vi "S3859061_Task4.vi"() -> ()   [LabVIEW 2020]
panel:
  out "String":string
  in  "Enum 2":enum16{"Pizza", "Fries", "Noodle"}(ring)
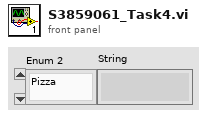
[diagram p1: front panel]
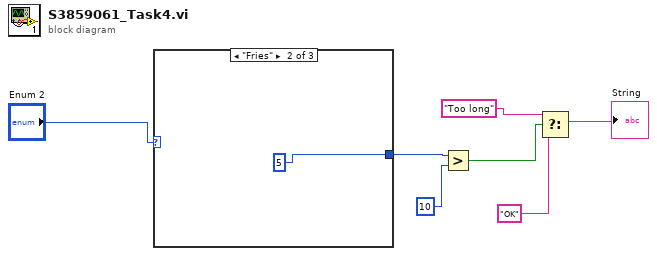
[diagram p0: block diagram]
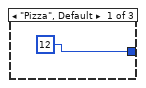
[diagram p2: hidden frame]
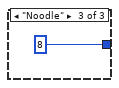
[diagram p3: hidden frame]
diagram:
  n1 = case shown="\"Fries\"" "Enum 2" {
    tunnel: [12 5 8] -> w6
    frame "Pizza", Default {
    }
    frame "Fries" {
    }
    frame "Noodle" {
    }
  }
  n2 = Greater?(x=w6, y=10) -> (0:w4:bool)
  n3 = Select(t="Too long", s=w4, f="OK") -> (s? t:f=→"String":string)
